vi "Util_AddSingleEmptyStringElementToZeroElementArray.vi"(1 "Array In":string[](array[string])) -> (0 "Array Out":string[](array[string]))   [LabVIEW 2014]
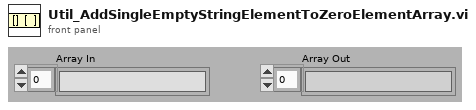
[diagram p1: front panel]
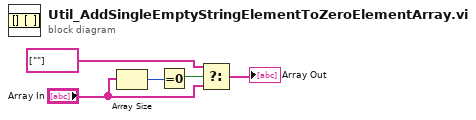
[diagram p0: block diagram]
diagram:
  n1 = Array Size(array="Array In") -> (size(s)=w1:i32)
  n2 = Equal To 0?(x=w1) -> (x = 0?=w2:bool)
  n3 = Select(t=string[] [""], s=w2, f="Array In") -> (s? t:f=→"Array Out":string[])
